vi "New Session SetUp.vi"(8 "error in (no error)":errorcluster, 10 "Stop Refnum":refnum<vi>, 11 "Generic Instrument in":refnum<class "Generic Instrument.lvclass">) -> (0 "error out":errorcluster, 3 "Generic Instrument out":refnum<class "Generic Instrument.lvclass">)   [LabVIEW 2014, in "Generic Instrument.lvlib" / "Generic Instrument.lvclass"]
uses:
  Generic Instrument.lvclass
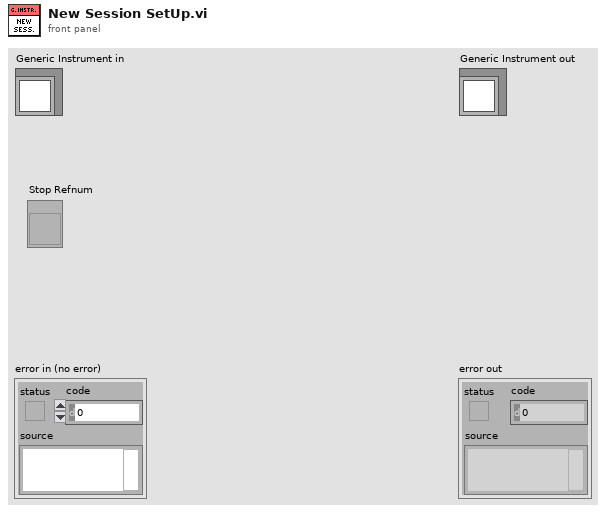
[diagram p1: front panel]
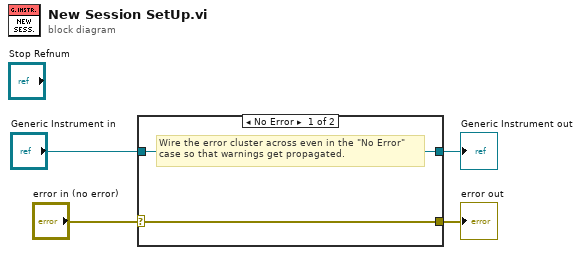
[diagram p0: block diagram]
diagram:
  n1 = case shown="No Error" "error in (no error)" {
    selector: "error in (no error)" -> [w5 w8]
    tunnel: [w5 w8] -> w3
    tunnel: [w6 w7] -> w1
    tunnel: "Generic Instrument in" -> [w6 w7]
    frame No Error {
      # "Wire the error cluster across even in the \"No Error\"\ncase so that warnings get propagated."
    }
    frame Error {
    }
  }
  "error out" <- w3
  "Generic Instrument out" <- w1
